vi "SR830ReadCalculateAverageInputsNoTimer.vi"(0 "VISA resource name":refnum<visa-resource-name>="SR830LockIn2", 3 "number of averaging points":i32=5, 5 "error in (no error)":errorcluster) -> (6 "R":dbl format="%0.3g", 7 "Temp (K)":dbl format="%0.3f", 8 "R-StDev":dbl format="%0.3g", 9 "Temp-StDev":dbl format="%0.3f", 10 "Theta (degrees)":dbl format="%0.3g", 12 "Theta-StDev (degrees)":dbl format="%0.3g", 14 "VISA resource name out":refnum<visa-resource-name>, 19 "error out":errorcluster)   [LabVIEW 2016]
uses:
  <vilib>/Analysis/NI_AALBase.lvlib
panel:
  # "This VI grabs input values simulatneously from the SR830, averages them anc caluclates the\nstandard deviation. The measurement time is measured and a bandwidth is calculated."
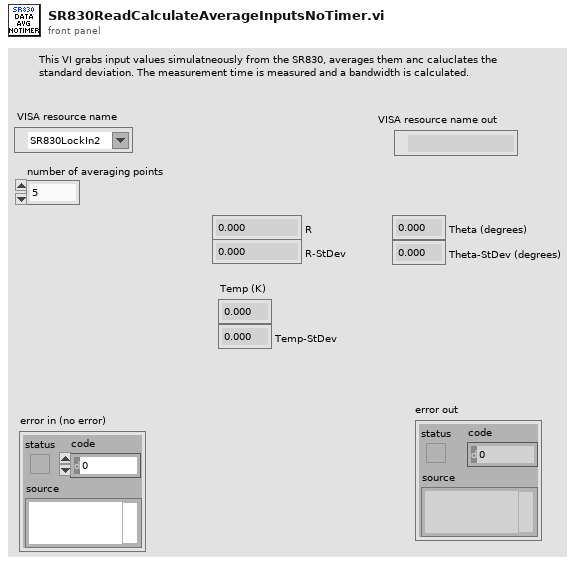
[diagram p1: front panel]
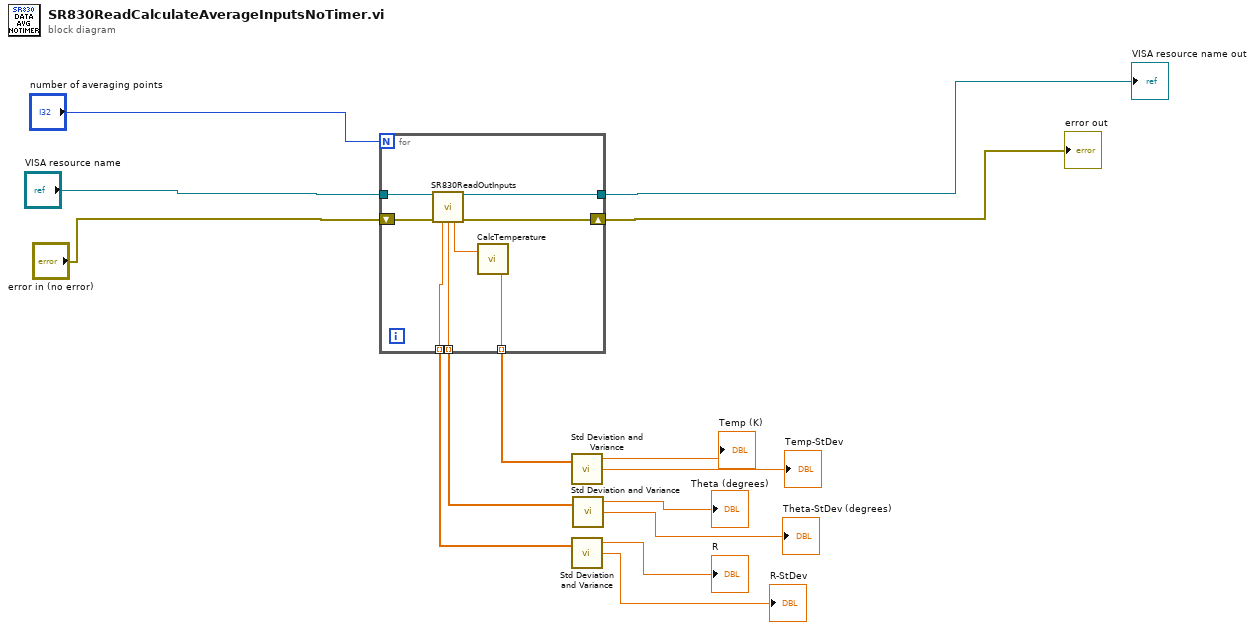
[diagram p0: block diagram]
diagram:
  n1 = for {
    N: "number of averaging points" -> [_]
    tunnel: "VISA resource name" -> [w21]
    tunnel: [w19] -> w11
    shift-right: [w18] -> w10
    shift-left: "error in (no error)" -> [w20]
    tunnel: [w17] -> w9 mode=indexing
    tunnel: [w16] -> w7 mode=indexing
    tunnel: [w15] -> w6 mode=indexing
    n2 = call "SR830ReadOutInputs.vi"("VISA resource name"=w21, "error in (no error)"=w20) -> ("VISA resource name out"=w19:refnum<visa-resource-name>, "R"=w15:dbl, "Theta"=w16:dbl, "Aux In 1"=w22:dbl, "error out"=w18:errorcluster)  [unwired: 9 in]
    n3 = call "CalcTemperature.vi"("Temp Voltage (V)"=w22) -> ("Temperature (K)"=w17:dbl)  [unwired: 1 in]
  }
  "VISA resource name out" <- w11
  "error out" <- w10
  n4 = call <vilib>:"Std Deviation and Variance.vi"("X"=w9) -> ("mean"=→"Temp (K)":dbl, "standard deviation"=→"Temp-StDev":dbl)  [unwired: 1 in, 1 out]
  n5 = call <vilib>:"Std Deviation and Variance.vi"("X"=w6) -> ("mean"=→"R":dbl, "standard deviation"=→"R-StDev":dbl)  [unwired: 1 in, 1 out]
  n6 = call <vilib>:"Std Deviation and Variance.vi"("X"=w7) -> ("mean"=→"Theta (degrees)":dbl, "standard deviation"=→"Theta-StDev (degrees)":dbl)  [unwired: 1 in, 1 out]
